vi "PointInPolygon.vi"(1 "Polygon":T1, 2 "2DPoint":T2) -> (0 "InPolygon":bool)   [LabVIEW 2018, in "ArgosLib.lvlib"]
uses:
  ArgosLib.lvlib
  TypeDefs/Point2D.ctl
  TypeDefs/Polygon2D.ctl
  <vilib>/Analysis/geometry.llb/Point in Polygon Position.ctl
  <vilib>/Analysis/geometry.llb/Point in Polygon (Scalar).vi
  <vilib>/Analysis/NI_AAL_Geometry.lvlib
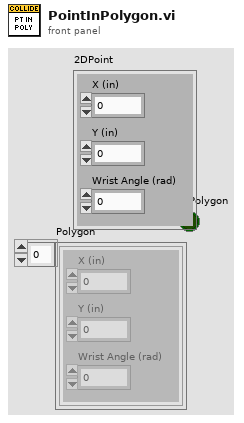
[diagram p1: front panel]
types:
  T1 = typedef "ArgosLib.lvlib/Polygon2D.ctl" = T2[]
  T2 = typedef "ArgosLib.lvlib/Point2D.ctl" = cluster{"X (in)":dbl, "Y (in)":dbl, "Wrist Angle (rad)":dbl}
  T3 = typedef "NI_AAL_Geometry.lvlib/Point in Polygon Position.ctl" = u16
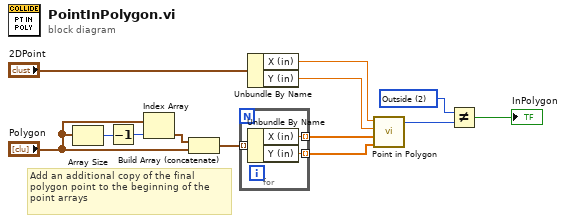
[diagram p0: block diagram]
diagram:
  w6 = T3 2 items=["Inside", "On Boundary", "Outside"] ("x")
  # "Add an additional copy of the final\npolygon point to the beginning of the\npoint arrays"
  n1 = Array Size(array="Polygon") -> (size(s)=w8:i32)
  n2 = Decrement(x=w8) -> (x-1=w11:i32)
  n3 = Index Array(array="Polygon", index=w11) -> (element=w9:T2)
  n4 = Build Array (concatenate)(w9, "Polygon") -> (w10:T1)
  n5 = for {
    tunnel: w10 -> [w16] mode=indexing
    tunnel: [w15] -> w4 mode=indexing
    tunnel: [w14] -> w3 mode=indexing
    n6 = Unbundle By Name(w16) -> ("X (in)"=w15:dbl, "Y (in)"=w14:dbl)
  }
  n7 = Unbundle By Name("2DPoint") -> ("X (in)"=w2:dbl, "Y (in)"=w1:dbl)
  n8 = call-poly <vilib>:"Point in Polygon.vi"("Polygon Y"=w3, "Polygon X"=w4, "y"=w1, "x"=w2) -> ("position"=w7:T3)  [unwired: 6 in, 1 out]
  n9 = Not Equal?(x=w6, y=w7) -> (x != y?=→"InPolygon":bool)
